vi "SendToAll.vi"(6 "Priority Message? (F)":bool, 8 "error in (no error)":errorcluster, 10 "Message":string, 11 "Message Queues in":T1) -> (0 "error out":errorcluster)   [LabVIEW 2017, in "Server.lvlib"]
uses:
  Server.lvlib
  SubLibs/Message Queue/CommReferences.ctl
  SubLibs/Message Queue/MessageCluster.ctl
  SubLibs/Message Queue/EnqueueMessage(Single).vi
  SubLibs/Message Queue/Message Queue.lvlib
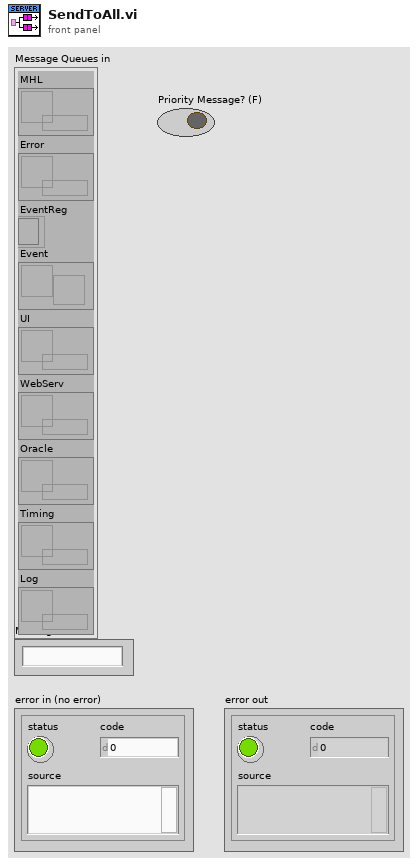
[diagram p1: front panel]
types:
  T1 = typedef "Server.lvlib/Message Queue.lvlib/CommReferences.ctl" = cluster{"MHL":refnum<queue>, "Error":refnum<queue>, "EventReg":refnum<event-registration>, "Event":refnum<user-event>, "UI":refnum<queue>, "WebServ":refnum<queue>, "Oracle":refnum<queue>, "Timing":refnum<queue>, "Log":refnum<queue>}
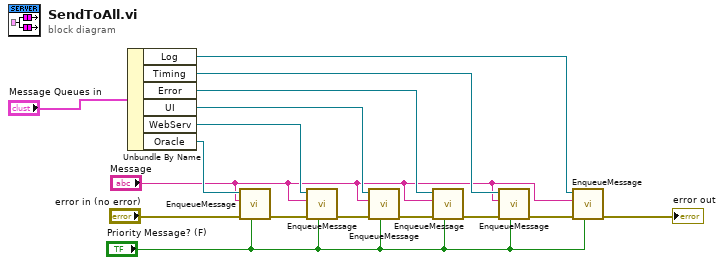
[diagram p0: block diagram]
diagram:
  n1 = Unbundle By Name("Message Queues in") -> ("Log"=w3:refnum<queue>, "Timing"=w16:refnum<queue>, "Error"=w14:refnum<queue>, "UI"=w13:refnum<queue>, "WebServ"=w12:refnum<queue>, "Oracle"=w11:refnum<queue>)
  n2 = call-poly "EnqueueMessage.vi"("Priority Message? (F)"="Priority Message? (F)", "error in (no error)"="error in (no error)", "Message"="Message", "Message Queue"=w11) -> ("error out"=w7:errorcluster)  [unwired: 6 in, 1 out]
  n3 = call-poly "EnqueueMessage.vi"("Priority Message? (F)"="Priority Message? (F)", "error in (no error)"=w7, "Message"="Message", "Message Queue"=w12) -> ("error out"=w8:errorcluster)  [unwired: 6 in, 1 out]
  n4 = call-poly "EnqueueMessage.vi"("Priority Message? (F)"="Priority Message? (F)", "error in (no error)"=w8, "Message"="Message", "Message Queue"=w13) -> ("error out"=w9:errorcluster)  [unwired: 6 in, 1 out]
  n5 = call-poly "EnqueueMessage.vi"("Priority Message? (F)"="Priority Message? (F)", "error in (no error)"=w9, "Message"="Message", "Message Queue"=w14) -> ("error out"=w15:errorcluster)  [unwired: 6 in, 1 out]
  n6 = call-poly "EnqueueMessage.vi"("Priority Message? (F)"="Priority Message? (F)", "error in (no error)"=w15, "Message"="Message", "Message Queue"=w16) -> ("error out"=w5:errorcluster)  [unwired: 6 in, 1 out]
  n7 = call-poly "EnqueueMessage.vi"("Priority Message? (F)"="Priority Message? (F)", "error in (no error)"=w5, "Message"="Message", "Message Queue"=w3) -> ("error out"=→"error out":errorcluster)  [unwired: 6 in, 1 out]
